vi "setMeasurement.vi"(8 "error in (no error)":errorcluster, 9 "conversion":T1, 10 "measurement":T2, 11 "Instrument.VSource in":refnum<class "Instrument.VNA.lvclass">) -> (0 "error out":errorcluster, 3 "Instrument.VSource out":refnum<class "Instrument.VNA.lvclass">)   [LabVIEW 2019, in "Instrument.VNA.lvclass"]
uses:
  Instrument.VNA.lvclass
  C:/Users/patrick/Documents/GitHub/Instrument-Framework/lvsrc/Instrument/Instrument.lvclass
  Typedefs/Measurement--enum.ctl
  Typedefs/Conversion--enum.ctl
  Typedefs/setMeasurement--cluster.ctl
  f1f1729c-74eb-4407-a9dc-4df0a687eb2b.vi
  f1f1729c-74eb-4407-a9dc-4df0a687eb2b.vi/55c127a8-29d1-46f0-bcf6-ee09619a4d87.vi
  f1f1729c-74eb-4407-a9dc-4df0a687eb2b.vi/55c127a8-29d1-46f0-bcf6-ee09619a4d87.vi/60c1efd0-6167-47ef-8ef3-69c7c2f36fd0.vi
  f1f1729c-74eb-4407-a9dc-4df0a687eb2b.vi/55c127a8-29d1-46f0-bcf6-ee09619a4d87.vi/d5cf0374-20ae-4942-9f70-82ff7617e098.vi
  Instrument/Private/Get RC Connection Status.vi
  Instrument/API/Send and Receive.vi
  <vilib>/Utility/Data Type/Get Type Information.vi
  <vilib>/JDP Science/JSONtext/JSON text to Variant.vi
  <vilib>/JDP Science/JSONtext/LVClass Serializer/JSONtext LVClass Serializer.lvclass
  Instrument/Instrument.lvclass
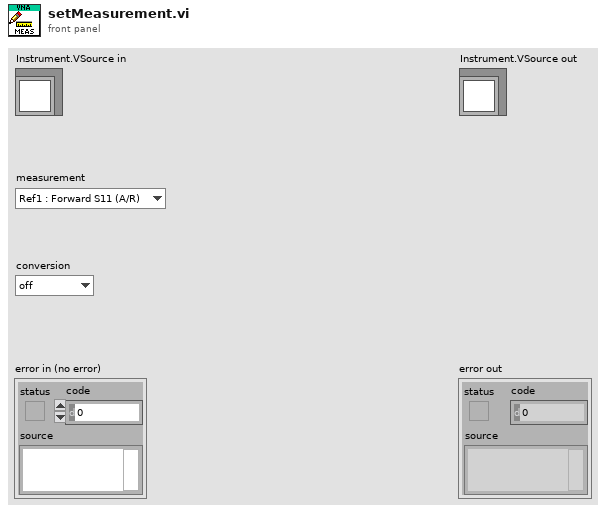
[diagram p1: front panel]
types:
  T1 = typedef "Instrument.VNA.lvclass/Conversion--enum.ctl" = enum16{"off", "Z: Ref1", "Z: Trans", "Y: Ref1", "Y: Trans", "1/S"}
  T2 = typedef "Instrument.VNA.lvclass/Measurement--enum.ctl" = enum16{"Ref1 : Forward S11 (A/R)", "Trans: Forward S21 (B/R)", "Trans: Reverse S12 (A/R)", "Ref1: Reverse S22 (B/R)", "Analog In, AUX input", "A/R", "B/R", "A/B", "A", "B", "R"}
  T3 = typedef "Instrument.VNA.lvclass/setMeasurement--cluster.ctl" = cluster{"measurement":T2, "conversion":T1}
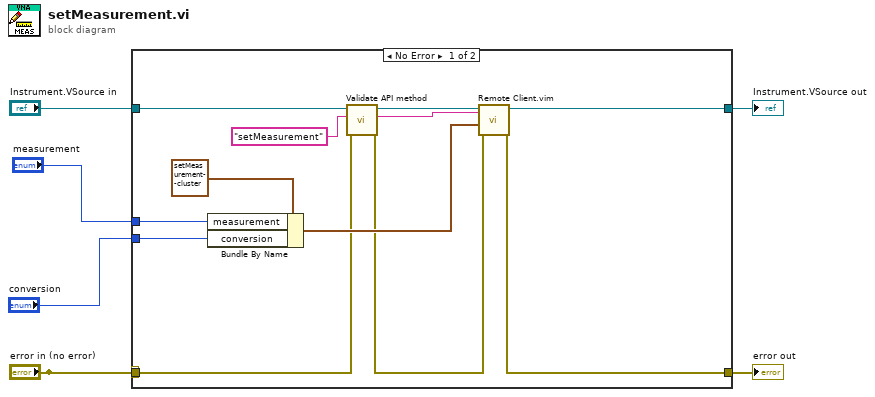
[diagram p0: block diagram]
diagram:
  n1 = case shown="No Error" "error in (no error)" {
    selector: "error in (no error)" -> [_ w20]
    tunnel: [w11 w20] -> w6
    tunnel: [w14 w19] -> w4
    tunnel: "Instrument.VSource in" -> [w15 w19]
    tunnel: "error in (no error)" -> [w13 _]
    tunnel: "measurement" -> [w9 _]
    tunnel: "conversion" -> [w8 _]
    frame No Error {
      n2 = Bundle By Name(cluster=T3 {"measurement"=enum."Ref1 : Forward S11 (A/R)", "conversion"=enum."off"} ("seConversion"), "measurement"=w9, "conversion"=w8) -> (w16:T3)
      n3 = call "Validate API method.vi"("error in (no error)"=w13, "Command in"="setMeasurement" ("error message (\"\")"), "Instrument in"=w15) -> ("error out"=w12:errorcluster, "command out"=w7:string, "Instrument out"=w17:refnum<class "Instrument.VNA.lvclass">)  [unwired: 6 in]
      n4 = call "Remote Client.vim"("Data Out type"=w7, "error in (no error)"=w12, "Data in"=w16, "Instrument in"=w17) -> ("error out"=w11:errorcluster, "Instrument out"=w14:refnum<class "Instrument.VNA.lvclass">)  [unwired: 4 in, 2 out]
    }
    frame Error {
    }
  }
  "error out" <- w6
  "Instrument.VSource out" <- w4
